vi "S4GUI_003.vi"(7 "Tab ObsEng":enum32{"Obs", "CCD modes", "Guider", "Eng"}(tab)) -> ()   [LabVIEW 2018] (continued)
                n3552 = call-dynamic "Read Interface.vi"("error in (no error)"=w7918, "Channel in"=w7920) -> ("error out"=w7931:errorcluster, "Interface.lvclass"=w7932:refnum<class "Interface.lvclass">, "Channel out"=w7944:refnum<class "Channel.lvclass">)  [unwired: 7 in]
                n3553 = call-dynamic "Write Suffix.vi"("error in (no error)"=w7931, "Suffix"=w7950, "Interface in"=w7932) -> ("error out"=w7949:errorcluster, "Interface out"=w7943:refnum<class "Interface.lvclass">)  [unwired: 7 in]
                n3554 = call-dynamic "Write ObsType.vi"("error in (no error)"=w7949, "ObsType"=w7935, "Interface in"=w7943) -> ("error out"=w7948:errorcluster, "Interface out"=w7942:refnum<class "Interface.lvclass">)  [unwired: 7 in]
                n3555 = call-dynamic "Write Object.vi"("error in (no error)"=w7948, "Object"=w7934, "Interface in"=w7942) -> ("error out"=w7947:errorcluster, "Interface out"=w7941:refnum<class "Interface.lvclass">)  [unwired: 7 in]
                n3556 = call-dynamic "Write Comments.vi"("error in (no error)"=w7947, "Comments"=w7936, "Interface in"=w7941) -> ("error out"=w7930:errorcluster, "Interface out"=w7929:refnum<class "Interface.lvclass">)  [unwired: 7 in]
                n3557 = call-dynamic "Write Observer.vi"("error in (no error)"=w7930, "Observer"=w7933, "Interface in"=w7929) -> ("error out"=w7928:errorcluster, "Interface out"=w7927:refnum<class "Interface.lvclass">)  [unwired: 7 in]
                n3558 = call-dynamic "Write Interface.vi"("error in (no error)"=w7928, "Interface.lvclass"=w7927, "Channel in"=w7944) -> ("error out"=w7924:errorcluster, "Channel out"=w7926:refnum<class "Channel.lvclass">)  [unwired: 7 in]
                n3559 = disable-structure shown="Enabled" {
                  disable-tunnel: w7926 -> [w7961 w7966]
                  disable-tunnel: [w7959 w7966] -> w7925
                  disable-tunnel: w7924 -> [w7958 w7965]
                  disable-tunnel: [w7957 w7965] -> w7923
                  frame Disabled {
                    n3560 = call-dynamic "Read State Machine.vi"("error in (no error)"=w7958, "Device in"=w7961) -> ("error out"=w7964:errorcluster, "State Machine.lvclass"=w7956:refnum<class "State Machine.lvclass">, "Device out"=w7960:refnum<class "Channel.lvclass">)  [unwired: 7 in]
                    n3561 = call "Next State.vi"("error in (no error)"=w7964, "New_State"=12, "State Machine in"=w7956) -> ("error out"=w7963:errorcluster, "State Machine out"=w7955:refnum<class "State Machine.lvclass">)  [unwired: 7 in]
                    n3562 = call-dynamic "Write State Machine.vi"("error in (no error)"=w7963, "State Machine.lvclass"=w7955, "Device in"=w7960) -> ("error out"=w7957:errorcluster, "Device out"=w7959:refnum<class "Channel.lvclass">)  [unwired: 7 in]
                  }
                  frame Enabled {
                  }
                }
                n3563 = call-dynamic "Write Channel.vi"("error in (no error)"=w7923, "Channel.lvclass"=w7925, "Acquisition in"=w7939) -> ("error out"=w7937:errorcluster, "Acquisition out"=w7938:refnum<class "Acquisition.lvclass">)  [unwired: 7 in]
                n3564 = call-dynamic "Write AcquisitionD.vi"("error in (no error)"=w7937, "Acquisition.lvclass"=w7938, "S4ACS_GUI in"=w7940) -> ("error out"=w7951:errorcluster, "S4ACS_GUI out"=w7952:refnum<class "S4GUI.lvclass">)  [unwired: 7 in]
              }
            }
          }
          frame True {
          }
        }
      }
      event "Observer": Mouse Enter {
        n3565 = event-data() -> ()  [unwired: 1 in, 4 out]
        n3566 = disable-structure shown="Disabled" {
          disable-tunnel: [w7974 w7977] -> w7970
          disable-tunnel: w7969 -> [w7972 w7977]
          frame Disabled {
            n3567 = property on="Observer" class="Str"() -> ("Value"=w7973:string)  [unwired: 2 in, 2 out]
            n3568 = String Length(string=w7973) -> (length=w7976:i32)
            n3569 = Equal To 0?(x=w7976) -> (x = 0?=w7975:bool)
            n3570 = property on="Observer" class="Str"(error in=w7972, "Caption.Visible"=w7975) -> (error out=w7974:errorcluster)  [unwired: 1 in, 1 out]
          }
          frame Enabled {
            # "Não se usa mais o texto de fundo\ndo controle \"Observer\""
          }
        }
      }
      event "Filter1", "Filter2", "Filter3", "Filter4": Value Change {
        n3571 = event-data() -> ()  [unwired: 1 in, 6 out]
        n3572 = stacked-sequence {
          seq-local: [w8008 _ _ _] -> [_ w8072 _ _]
          seq-local: [w8007 _ _ _] -> [_ w8071 _ _]
          seq-local: [_ w8070 _ _] -> [_ _ w8121 _]
          seq-local: [_ w8069 _ _] -> [_ _ w8120 _]
          seq-local: [_ _ w8119 _] -> [_ _ _ w8170]
          seq-local: [_ _ w8118 _] -> [_ _ _ w8169]
          tunnel: w7985 -> [w8020 _ _ _]
          tunnel: w7986 -> [w8019 _ _ _]
          tunnel: [_ _ _ w8168] -> w7979
          tunnel: [_ _ _ w8167] -> w7978
          tunnel: w7983 -> [w8006 w8068 w8117 w8166]
          tunnel: w7982 -> [w8005 w8067 w8103 w8152]
          tunnel: w7980 -> [w8004 w8053 w8102 w8151]
          tunnel: w7984 -> [w8003 w8052 w8101 w8150]
          tunnel: w7981 -> [w8002 w8051 w8100 w8149]
          frame #0 {
            # "observer"
            # "comment"
            # "object"
            # "suffix"
            # "obsType"
            n3573 = call-dynamic "Read AcquisitionA.vi"("error in (no error)"=w8020, "S4ACS_GUI in"=w8019) -> ("error out"=w8018:errorcluster, "Acquisition.lvclass"=w8017:refnum<class "Acquisition.lvclass">, "S4ACS_GUI out"=w8012:refnum<class "S4GUI.lvclass">)  [unwired: 7 in]
            n3574 = call-dynamic "Read Channel.vi"("error in (no error)"=w8018, "Acquisition in"=w8017) -> ("error out"=w7988:errorcluster, "Channel.lvclass"=w7991:refnum<class "Channel.lvclass">, "Acquisition out"=w8011:refnum<class "Acquisition.lvclass">)  [unwired: 7 in]
            n3575 = local read "Filter1"() -> (w7989:u8)
            n3576 = call-dynamic "Write Filter.vi"("error in (no error)"=w7988, "Filter"=w7989, "Channel in"=w7991) -> ("error out"=w7987:errorcluster, "Channel out"=w7990:refnum<class "Channel.lvclass">)  [unwired: 7 in]
            n3577 = call-dynamic "Read Interface.vi"("error in (no error)"=w7987, "Channel in"=w7990) -> ("error out"=w7998:errorcluster, "Interface.lvclass"=w7999:refnum<class "Interface.lvclass">, "Channel out"=w8016:refnum<class "Channel.lvclass">)  [unwired: 7 in]
            n3578 = call-dynamic "Write Suffix.vi"("error in (no error)"=w7998, "Suffix"=w8006, "Interface in"=w7999) -> ("error out"=w8023:errorcluster, "Interface out"=w8015:refnum<class "Interface.lvclass">)  [unwired: 7 in]
            n3579 = call-dynamic "Write ObsType.vi"("error in (no error)"=w8023, "ObsType"=w8004, "Interface in"=w8015) -> ("error out"=w8022:errorcluster, "Interface out"=w8014:refnum<class "Interface.lvclass">)  [unwired: 7 in]
            n3580 = call-dynamic "Write Object.vi"("error in (no error)"=w8022, "Object"=w8003, "Interface in"=w8014) -> ("error out"=w8021:errorcluster, "Interface out"=w8013:refnum<class "Interface.lvclass">)  [unwired: 7 in]
            n3581 = call-dynamic "Write Comments.vi"("error in (no error)"=w8021, "Comments"=w8005, "Interface in"=w8013) -> ("error out"=w8001:errorcluster, "Interface out"=w8000:refnum<class "Interface.lvclass">)  [unwired: 7 in]
            n3582 = call-dynamic "Write Observer.vi"("error in (no error)"=w8001, "Observer"=w8002, "Interface in"=w8000) -> ("error out"=w7996:errorcluster, "Interface out"=w7997:refnum<class "Interface.lvclass">)  [unwired: 7 in]
            n3583 = call-dynamic "Write Interface.vi"("error in (no error)"=w7996, "Interface.lvclass"=w7997, "Channel in"=w8016) -> ("error out"=w7993:errorcluster, "Channel out"=w7995:refnum<class "Channel.lvclass">)  [unwired: 7 in]
            n3584 = disable-structure shown="Enabled" {
              disable-tunnel: w7995 -> [w8033 w8035]
              disable-tunnel: [w8031 w8035] -> w7994
              disable-tunnel: w7993 -> [w8030 w8034]
              disable-tunnel: [w8025 w8034] -> w7992
              frame Disabled {
                n3585 = call-dynamic "Read State Machine.vi"("error in (no error)"=w8030, "Device in"=w8033) -> ("error out"=w8029:errorcluster, "State Machine.lvclass"=w8027:refnum<class "State Machine.lvclass">, "Device out"=w8032:refnum<class "Channel.lvclass">)  [unwired: 7 in]
                n3586 = call "Next State.vi"("error in (no error)"=w8029, "New_State"=12, "State Machine in"=w8027) -> ("error out"=w8028:errorcluster, "State Machine out"=w8026:refnum<class "State Machine.lvclass">)  [unwired: 7 in]
                n3587 = call-dynamic "Write State Machine.vi"("error in (no error)"=w8028, "State Machine.lvclass"=w8026, "Device in"=w8032) -> ("error out"=w8025:errorcluster, "Device out"=w8031:refnum<class "Channel.lvclass">)  [unwired: 7 in]
              }
              frame Enabled {
              }
            }
            n3588 = call-dynamic "Write Channel.vi"("error in (no error)"=w7992, "Channel.lvclass"=w7994, "Acquisition in"=w8011) -> ("error out"=w8009:errorcluster, "Acquisition out"=w8010:refnum<class "Acquisition.lvclass">)  [unwired: 7 in]
            n3589 = call-dynamic "Write AcquisitionA.vi"("error in (no error)"=w8009, "Acquisition.lvclass"=w8010, "S4ACS_GUI in"=w8012) -> ("error out"=w8007:errorcluster, "S4ACS_GUI out"=w8008:refnum<class "S4GUI.lvclass">)  [unwired: 7 in]
          }
          frame #1 {
            # "object"
            # "suffix"
            # "obsType"
            n3590 = call "Read AcquisitionB.vi"("error in (no error)"=w8071, "S4ACS_GUI in"=w8072) -> ("error out"=w8057:errorcluster, "Acquisition.lvclass"=w8058:refnum<class "Acquisition.lvclass">, "S4ACS_GUI out"=w8063:refnum<class "S4GUI.lvclass">)  [unwired: 7 in]
            n3591 = call-dynamic "Read Channel.vi"("error in (no error)"=w8057, "Acquisition in"=w8058) -> ("error out"=w8037:errorcluster, "Channel.lvclass"=w8039:refnum<class "Channel.lvclass">, "Acquisition out"=w8064:refnum<class "Acquisition.lvclass">)  [unwired: 7 in]
            n3592 = local read "Filter2"() -> (w8040:u8)
            n3593 = call-dynamic "Write Filter.vi"("error in (no error)"=w8037, "Filter"=w8040, "Channel in"=w8039) -> ("error out"=w8036:errorcluster, "Channel out"=w8038:refnum<class "Channel.lvclass">)  [unwired: 7 in]
            n3594 = call-dynamic "Read Interface.vi"("error in (no error)"=w8036, "Channel in"=w8038) -> ("error out"=w8045:errorcluster, "Interface.lvclass"=w8046:refnum<class "Interface.lvclass">, "Channel out"=w8059:refnum<class "Channel.lvclass">)  [unwired: 7 in]
            n3595 = call-dynamic "Write Suffix.vi"("error in (no error)"=w8045, "Suffix"=w8068, "Interface in"=w8046) -> ("error out"=w8054:errorcluster, "Interface out"=w8060:refnum<class "Interface.lvclass">)  [unwired: 7 in]
            n3596 = call-dynamic "Write ObsType.vi"("error in (no error)"=w8054, "ObsType"=w8053, "Interface in"=w8060) -> ("error out"=w8055:errorcluster, "Interface out"=w8061:refnum<class "Interface.lvclass">)  [unwired: 7 in]
            n3597 = call-dynamic "Write Object.vi"("error in (no error)"=w8055, "Object"=w8052, "Interface in"=w8061) -> ("error out"=w8056:errorcluster, "Interface out"=w8062:refnum<class "Interface.lvclass">)  [unwired: 7 in]
            n3598 = call-dynamic "Write Comments.vi"("error in (no error)"=w8056, "Comments"=w8067, "Interface in"=w8062) -> ("error out"=w8048:errorcluster, "Interface out"=w8047:refnum<class "Interface.lvclass">)  [unwired: 7 in]
            n3599 = call-dynamic "Write Observer.vi"("error in (no error)"=w8048, "Observer"=w8051, "Interface in"=w8047) -> ("error out"=w8049:errorcluster, "Interface out"=w8050:refnum<class "Interface.lvclass">)  [unwired: 7 in]
            n3600 = call-dynamic "Write Interface.vi"("error in (no error)"=w8049, "Interface.lvclass"=w8050, "Channel in"=w8059) -> ("error out"=w8043:errorcluster, "Channel out"=w8044:refnum<class "Channel.lvclass">)  [unwired: 7 in]
            n3601 = disable-structure shown="Enabled" {
              disable-tunnel: w8044 -> [w8077 w8084]
              disable-tunnel: w8043 -> [w8076 w8083]
              disable-tunnel: [w8074 w8084] -> w8042
              disable-tunnel: [w8073 w8083] -> w8041
              frame Disabled {
                n3602 = call-dynamic "Read State Machine.vi"("error in (no error)"=w8076, "Device in"=w8077) -> ("error out"=w8082:errorcluster, "State Machine.lvclass"=w8080:refnum<class "State Machine.lvclass">, "Device out"=w8075:refnum<class "Channel.lvclass">)  [unwired: 7 in]
                n3603 = call "Next State.vi"("error in (no error)"=w8082, "New_State"=12, "State Machine in"=w8080) -> ("error out"=w8081:errorcluster, "State Machine out"=w8079:refnum<class "State Machine.lvclass">)  [unwired: 7 in]
                n3604 = call-dynamic "Write State Machine.vi"("error in (no error)"=w8081, "State Machine.lvclass"=w8079, "Device in"=w8075) -> ("error out"=w8073:errorcluster, "Device out"=w8074:refnum<class "Channel.lvclass">)  [unwired: 7 in]
              }
              frame Enabled {
              }
            }
            n3605 = call-dynamic "Write Channel.vi"("error in (no error)"=w8041, "Channel.lvclass"=w8042, "Acquisition in"=w8064) -> ("error out"=w8066:errorcluster, "Acquisition out"=w8065:refnum<class "Acquisition.lvclass">)  [unwired: 7 in]
            n3606 = call "Write AcquisitionB.vi"("error in (no error)"=w8066, "Acquisition.lvclass"=w8065, "S4ACS_GUI in"=w8063) -> ("error out"=w8069:errorcluster, "S4ACS_GUI out"=w8070:refnum<class "S4GUI.lvclass">)  [unwired: 7 in]
          }
          frame #2 {
            # "object"
            # "suffix"
            # "obsType"
            n3607 = call-dynamic "Read AcquisitionC.vi"("error in (no error)"=w8120, "S4ACS_GUI in"=w8121) -> ("error out"=w8113:errorcluster, "Acquisition.lvclass"=w8112:refnum<class "Acquisition.lvclass">, "S4ACS_GUI out"=w8107:refnum<class "S4GUI.lvclass">)  [unwired: 7 in]
            n3608 = call-dynamic "Read Channel.vi"("error in (no error)"=w8113, "Acquisition in"=w8112) -> ("error out"=w8087:errorcluster, "Channel.lvclass"=w8089:refnum<class "Channel.lvclass">, "Acquisition out"=w8106:refnum<class "Acquisition.lvclass">)  [unwired: 7 in]
            n3609 = local read "Filter3"() -> (w8090:u8)
            n3610 = call-dynamic "Write Filter.vi"("error in (no error)"=w8087, "Filter"=w8090, "Channel in"=w8089) -> ("error out"=w8086:errorcluster, "Channel out"=w8088:refnum<class "Channel.lvclass">)  [unwired: 7 in]
            n3611 = call-dynamic "Read Interface.vi"("error in (no error)"=w8086, "Channel in"=w8088) -> ("error out"=w8098:errorcluster, "Interface.lvclass"=w8099:refnum<class "Interface.lvclass">, "Channel out"=w8111:refnum<class "Channel.lvclass">)  [unwired: 7 in]
            n3612 = call-dynamic "Write Suffix.vi"("error in (no error)"=w8098, "Suffix"=w8117, "Interface in"=w8099) -> ("error out"=w8116:errorcluster, "Interface out"=w8110:refnum<class "Interface.lvclass">)  [unwired: 7 in]
            n3613 = call-dynamic "Write ObsType.vi"("error in (no error)"=w8116, "ObsType"=w8102, "Interface in"=w8110) -> ("error out"=w8115:errorcluster, "Interface out"=w8109:refnum<class "Interface.lvclass">)  [unwired: 7 in]
            n3614 = call-dynamic "Write Object.vi"("error in (no error)"=w8115, "Object"=w8101, "Interface in"=w8109) -> ("error out"=w8114:errorcluster, "Interface out"=w8108:refnum<class "Interface.lvclass">)  [unwired: 7 in]
            n3615 = call-dynamic "Write Comments.vi"("error in (no error)"=w8114, "Comments"=w8103, "Interface in"=w8108) -> ("error out"=w8095:errorcluster, "Interface out"=w8094:refnum<class "Interface.lvclass">)  [unwired: 7 in]
            n3616 = call-dynamic "Write Observer.vi"("error in (no error)"=w8095, "Observer"=w8100, "Interface in"=w8094) -> ("error out"=w8096:errorcluster, "Interface out"=w8097:refnum<class "Interface.lvclass">)  [unwired: 7 in]
            n3617 = call-dynamic "Write Interface.vi"("error in (no error)"=w8096, "Interface.lvclass"=w8097, "Channel in"=w8111) -> ("error out"=w8092:errorcluster, "Channel out"=w8093:refnum<class "Channel.lvclass">)  [unwired: 7 in]
            n3618 = disable-structure shown="Enabled" {
              disable-tunnel: w8093 -> [w8128 w8133]
              disable-tunnel: w8092 -> [w8127 w8132]
              disable-tunnel: [w8122 w8132] -> w8091
              disable-tunnel: [w8125 w8133] -> w8085
              frame Disabled {
                n3619 = call-dynamic "Read State Machine.vi"("error in (no error)"=w8127, "Device in"=w8128) -> ("error out"=w8131:errorcluster, "State Machine.lvclass"=w8124:refnum<class "State Machine.lvclass">, "Device out"=w8126:refnum<class "Channel.lvclass">)  [unwired: 7 in]
                n3620 = call "Next State.vi"("error in (no error)"=w8131, "New_State"=12, "State Machine in"=w8124) -> ("error out"=w8130:errorcluster, "State Machine out"=w8123:refnum<class "State Machine.lvclass">)  [unwired: 7 in]
                n3621 = call-dynamic "Write State Machine.vi"("error in (no error)"=w8130, "State Machine.lvclass"=w8123, "Device in"=w8126) -> ("error out"=w8122:errorcluster, "Device out"=w8125:refnum<class "Channel.lvclass">)  [unwired: 7 in]
              }
              frame Enabled {
              }
            }
            n3622 = call-dynamic "Write Channel.vi"("error in (no error)"=w8091, "Channel.lvclass"=w8085, "Acquisition in"=w8106) -> ("error out"=w8104:errorcluster, "Acquisition out"=w8105:refnum<class "Acquisition.lvclass">)  [unwired: 7 in]
            n3623 = call-dynamic "Write AcquisitionC.vi"("error in (no error)"=w8104, "Acquisition.lvclass"=w8105, "S4ACS_GUI in"=w8107) -> ("error out"=w8118:errorcluster, "S4ACS_GUI out"=w8119:refnum<class "S4GUI.lvclass">)  [unwired: 7 in]
          }
          frame #3 {
            # "object"
            # "suffix"
            # "obsType"
            n3624 = call-dynamic "Read AcquisitionD.vi"("error in (no error)"=w8169, "S4ACS_GUI in"=w8170) -> ("error out"=w8162:errorcluster, "Acquisition.lvclass"=w8161:refnum<class "Acquisition.lvclass">, "S4ACS_GUI out"=w8156:refnum<class "S4GUI.lvclass">)  [unwired: 7 in]
            n3625 = call-dynamic "Read Channel.vi"("error in (no error)"=w8162, "Acquisition in"=w8161) -> ("error out"=w8135:errorcluster, "Channel.lvclass"=w8137:refnum<class "Channel.lvclass">, "Acquisition out"=w8155:refnum<class "Acquisition.lvclass">)  [unwired: 7 in]
            n3626 = local read "Filter4"() -> (w8138:u8)
            n3627 = call-dynamic "Write Filter.vi"("error in (no error)"=w8135, "Filter"=w8138, "Channel in"=w8137) -> ("error out"=w8134:errorcluster, "Channel out"=w8136:refnum<class "Channel.lvclass">)  [unwired: 7 in]
            n3628 = call-dynamic "Read Interface.vi"("error in (no error)"=w8134, "Channel in"=w8136) -> ("error out"=w8147:errorcluster, "Interface.lvclass"=w8148:refnum<class "Interface.lvclass">, "Channel out"=w8160:refnum<class "Channel.lvclass">)  [unwired: 7 in]
            n3629 = call-dynamic "Write Suffix.vi"("error in (no error)"=w8147, "Suffix"=w8166, "Interface in"=w8148) -> ("error out"=w8165:errorcluster, "Interface out"=w8159:refnum<class "Interface.lvclass">)  [unwired: 7 in]
            n3630 = call-dynamic "Write ObsType.vi"("error in (no error)"=w8165, "ObsType"=w8151, "Interface in"=w8159) -> ("error out"=w8164:errorcluster, "Interface out"=w8158:refnum<class "Interface.lvclass">)  [unwired: 7 in]
            n3631 = call-dynamic "Write Object.vi"("error in (no error)"=w8164, "Object"=w8150, "Interface in"=w8158) -> ("error out"=w8163:errorcluster, "Interface out"=w8157:refnum<class "Interface.lvclass">)  [unwired: 7 in]
            n3632 = call-dynamic "Write Comments.vi"("error in (no error)"=w8163, "Comments"=w8152, "Interface in"=w8157) -> ("error out"=w8146:errorcluster, "Interface out"=w8145:refnum<class "Interface.lvclass">)  [unwired: 7 in]
            n3633 = call-dynamic "Write Observer.vi"("error in (no error)"=w8146, "Observer"=w8149, "Interface in"=w8145) -> ("error out"=w8144:errorcluster, "Interface out"=w8143:refnum<class "Interface.lvclass">)  [unwired: 7 in]
            n3634 = call-dynamic "Write Interface.vi"("error in (no error)"=w8144, "Interface.lvclass"=w8143, "Channel in"=w8160) -> ("error out"=w8140:errorcluster, "Channel out"=w8142:refnum<class "Channel.lvclass">)  [unwired: 7 in]
            n3635 = disable-structure shown="Enabled" {
              disable-tunnel: w8142 -> [w8177 w8182]
              disable-tunnel: [w8175 w8182] -> w8141
              disable-tunnel: w8140 -> [w8174 w8181]
              disable-tunnel: [w8173 w8181] -> w8139
              frame Disabled {
                n3636 = call-dynamic "Read State Machine.vi"("error in (no error)"=w8174, "Device in"=w8177) -> ("error out"=w8180:errorcluster, "State Machine.lvclass"=w8172:refnum<class "State Machine.lvclass">, "Device out"=w8176:refnum<class "Channel.lvclass">)  [unwired: 7 in]
                n3637 = call "Next State.vi"("error in (no error)"=w8180, "New_State"=12, "State Machine in"=w8172) -> ("error out"=w8179:errorcluster, "State Machine out"=w8171:refnum<class "State Machine.lvclass">)  [unwired: 7 in]
                n3638 = call-dynamic "Write State Machine.vi"("error in (no error)"=w8179, "State Machine.lvclass"=w8171, "Device in"=w8176) -> ("error out"=w8173:errorcluster, "Device out"=w8175:refnum<class "Channel.lvclass">)  [unwired: 7 in]
              }
              frame Enabled {
              }
            }
            n3639 = call-dynamic "Write Channel.vi"("error in (no error)"=w8139, "Channel.lvclass"=w8141, "Acquisition in"=w8155) -> ("error out"=w8153:errorcluster, "Acquisition out"=w8154:refnum<class "Acquisition.lvclass">)  [unwired: 7 in]
            n3640 = call-dynamic "Write AcquisitionD.vi"("error in (no error)"=w8153, "Acquisition.lvclass"=w8154, "S4ACS_GUI in"=w8156) -> ("error out"=w8167:errorcluster, "S4ACS_GUI out"=w8168:refnum<class "S4GUI.lvclass">)  [unwired: 7 in]
          }
        }
      }
      event "Start ch1": Value Change {
        n3641 = event-data() -> ()  [unwired: 1 in, 6 out]
        n3642 = call "Read Instrument.lvclass.vi"("error in (no error)"=w8195, "S4ACS_GUI in"=w8197) -> ("error out"=w8198:errorcluster, "Instrument.lvclass"=w8199:refnum<class "Instrument.lvclass">, "S4ACS_GUI out"=w8196:refnum<class "S4GUI.lvclass">)  [unwired: 7 in]
        n3643 = call-dynamic "Read mode.vi"("error in (no error)"=w8198, "Instrument in"=w8199) -> ("error out"=w8194:errorcluster, "mode"=w8193:bool)  [unwired: 7 in, 1 out]
        n3644 = call-dynamic "Read AcquisitionA.vi"("error in (no error)"=w8194, "S4ACS_GUI in"=w8196) -> ("error out"=w8211:errorcluster, "Acquisition.lvclass"=w8212:refnum<class "Acquisition.lvclass">, "S4ACS_GUI out"=w8214:refnum<class "S4GUI.lvclass">)  [unwired: 7 in]
        n3645 = call-dynamic "Read Acq_state.vi"("error in (no error)"=w8211, "Acquisition in"=w8212) -> ("error out"=w8208:errorcluster, "Acq_state"=w8210:u32, "Acquisition out"=w8207:refnum<class "Acquisition.lvclass">)  [unwired: 7 in]
        n3646 = Not Equal?(x=w8210, y=u32 400) -> (x != y?=w8213:bool)
        n3647 = case shown="True" w8213 {
          tunnel: w8214 -> [w8227 w8266]
          tunnel: [w8227 w8257] -> w8206
          tunnel: [w8222 w8247] -> w8192
          tunnel: w8208 -> [w8229 w8260]
          tunnel: w8207 -> [w8232 w8256]
          tunnel: [w8223 w8248] -> w8205
          tunnel: w8204 -> [_ w8279]
          tunnel: w8203 -> [_ w8278]
          tunnel: w8202 -> [_ w8277]
          tunnel: w8201 -> [_ w8276]
          tunnel: w8200 -> [_ w8271]
          tunnel: w8193 -> [_ _]
          tunnel: w8191 -> [_ w8251]
          tunnel: w8190 -> [_ w8254]
          tunnel: w8189 -> [_ w8253]
          tunnel: w8188 -> [_ w8252]
          frame False {
            n3648 = call-dynamic "Read Acq_prevstate.vi"("error in (no error)"=w8229, "Acquisition in"=w8232) -> ("error out"=w8228:errorcluster, "Acq_prevstate"=w8230:u32, "Acquisition out"=w8231:refnum<class "Acquisition.lvclass">)  [unwired: 7 in]
            n3649 = call-dynamic "Write Acq_state.vi"("error in (no error)"=w8228, "Acq_state"=w8230, "Acquisition in"=w8231) -> ("error out"=w8219:errorcluster, "Acquisition out"=w8221:refnum<class "Acquisition.lvclass">)  [unwired: 7 in]
            n3650 = call-dynamic "Read enabled.vi"("error in (no error)"=w8219, "Server in"=w8221) -> ("error out"=w8218:errorcluster, "enabled"=w8215:bool, "Server out"=w8220:refnum<class "Acquisition.lvclass">)  [unwired: 7 in]
            n3651 = call-dynamic "Read Channel.vi"("error in (no error)"=w8218, "Acquisition in"=w8220) -> ("error out"=w8216:errorcluster, "Channel.lvclass"=w8217:refnum<class "Channel.lvclass">, "Acquisition out"=w8226:refnum<class "Acquisition.lvclass">)  [unwired: 7 in]
            n3652 = case shown="True" w8215 {
              tunnel: w8217 -> [w8234 w8244]
              tunnel: [w8234 w8242] -> w8225
              tunnel: w8216 -> [w8233 w8239]
              tunnel: [w8233 w8237] -> w8224
              frame False {
              }
              frame True {
                n3653 = call-dynamic "Read State Machine.vi"("error in (no error)"=w8239, "Device in"=w8244) -> ("error out"=w8235:errorcluster, "State Machine.lvclass"=w8236:refnum<class "State Machine.lvclass">, "Device out"=w8243:refnum<class "Channel.lvclass">)  [unwired: 7 in]
                n3654 = call "Next State.vi"("error in (no error)"=w8235, "New_State"=96, "State Machine in"=w8236) -> ("error out"=w8238:errorcluster, "State Machine out"=w8241:refnum<class "State Machine.lvclass">)  [unwired: 7 in]
                n3655 = call-dynamic "Write State Machine.vi"("error in (no error)"=w8238, "State Machine.lvclass"=w8241, "Device in"=w8243) -> ("error out"=w8237:errorcluster, "Device out"=w8242:refnum<class "Channel.lvclass">)  [unwired: 7 in]
              }
            }
            n3656 = call-dynamic "Write Channel.vi"("error in (no error)"=w8224, "Channel.lvclass"=w8225, "Acquisition in"=w8226) -> ("error out"=w8222:errorcluster, "Acquisition out"=w8223:refnum<class "Acquisition.lvclass">)  [unwired: 7 in]
          }
          frame True {
            # "vide S4GUI:\nHandleObservationAsync.vi"
            # "object"
            # "suffix"
            # "obsType"
            n3657 = call "Read Instrument.lvclass.vi"("S4ACS_GUI in"=w8266) -> ("error out"=w8268:errorcluster, "Instrument.lvclass"=w8270:refnum<class "Instrument.lvclass">, "S4ACS_GUI out"=w8258:refnum<class "S4GUI.lvclass">)  [unwired: 8 in]
            n3658 = call "Read WPROT.vi"("error in (no error)"=w8268, "Instrument in"=w8270) -> ("error out"=w8267:errorcluster, "Opt_Selector.lvclass"=w8269:refnum<class "Opt_Selector.lvclass">)  [unwired: 7 in, 1 out]
            n3659 = call-dynamic "Read sequencia.vi"("error in (no error)"=w8267, "Opt_Selector in"=w8269) -> ()  [unwired: 7 in, 3 out]
            n3660 = case shown="\"FOCUS\"" w8251 {
              tunnel: [u32 271 ("Obs_state") u32 251 ("Obs_state")] -> w8259
              tunnel: w8260 -> [w8302 w8313]
              tunnel: [w8301 w8313] -> w8255
              tunnel: w8254 -> [w8309 _]
              tunnel: w8253 -> [w8308 _]
              tunnel: w8252 -> [w8307 _]
              tunnel: w8258 -> [w8300 w8312]
              tunnel: [w8299 w8312] -> w8257
              frame "FOCUS" {
                n3661 = call-dynamic "Read TelFocus.lvclass.vi"("error in (no error)"=w8302, "S4GUI in"=w8300) -> ("error out"=w8304:errorcluster, "TelFocus.lvclass"=w8306:refnum<class "TelFocus.lvclass">, "S4GUI out"=w8310:refnum<class "S4GUI.lvclass">)  [unwired: 7 in]
                n3662 = call-dynamic "LoadParam.vi"("#steps"=w8307, "error in (no error)"=w8304, "step"=w8308, "init"=w8309, "TelFocus in"=w8306) -> ("error out"=w8303:errorcluster, "TelFocus out"=w8305:refnum<class "TelFocus.lvclass">)  [unwired: 5 in]
                n3663 = call-dynamic "Write TelFocus.lvclass.vi"("error in (no error)"=w8303, "TelFocus.lvclass"=w8305, "S4GUI in"=w8310) -> ("error out"=w8301:errorcluster, "S4GUI out"=w8299:refnum<class "S4GUI.lvclass">)  [unwired: 7 in]
              }
              frame Default {
              }
            }
            n3664 = property on="Start ch1" class="Bool"(error in=w8260, "DisabledEnum"=T12."Disabled and Grayed Out" ("Disabled")) -> ()  [unwired: 1 in, 2 out]
            n3665 = call-dynamic "Write Acq_state.vi"("error in (no error)"=w8255, "Acq_state"=w8259, "Acquisition in"=w8256) -> ("error out"=w8280:errorcluster, "Acquisition out"=w8281:refnum<class "Acquisition.lvclass">)  [unwired: 7 in]
            n3666 = call-dynamic "Read Channel.vi"("error in (no error)"=w8280, "Acquisition in"=w8281) -> ("error out"=w8282:errorcluster, "Channel.lvclass"=w8283:refnum<class "Channel.lvclass">, "Acquisition out"=w8287:refnum<class "Acquisition.lvclass">)  [unwired: 7 in]
            n3667 = call-dynamic "Read Interface.vi"("error in (no error)"=w8282, "Channel in"=w8283) -> ("error out"=w8297:errorcluster, "Interface.lvclass"=w8298:refnum<class "Interface.lvclass">, "Channel out"=w8296:refnum<class "Channel.lvclass">)  [unwired: 7 in]
            n3668 = call "Write Exposure Time.vi"("error in (no error)"=w8297, "Exposure Time"="Exptime ch1", "Interface in"=w8298) -> ("error out"=w8264:errorcluster, "Interface out"=w8265:refnum<class "Interface.lvclass">)  [unwired: 7 in]
            n3669 = case shown="Default" w8251 {
              tunnel: w8265 -> [w8316 w8321]
              tunnel: w8264 -> [w8315 w8320]
              tunnel: "Exptime ch1" -> [_ w8319]
              tunnel: [w8315 w8318] -> w8262
              tunnel: [w8316 w8317] -> w8261
              frame "ZERO" {
              }
              frame Default {
                n3670 = call-dynamic "Write prev ExpTime.vi"("error in (no error)"=w8320, "prev ExpTime"=w8319, "Interface in"=w8321) -> ("error out"=w8318:errorcluster, "Interface out"=w8317:refnum<class "Interface.lvclass">)  [unwired: 7 in]
              }
            }
            n3671 = call-dynamic "Write Suffix.vi"("error in (no error)"=w8262, "Suffix"=w8279, "Interface in"=w8261) -> ("error out"=w8295:errorcluster, "Interface out"=w8294:refnum<class "Interface.lvclass">)  [unwired: 7 in]
            n3672 = call-dynamic "Write ObsType.vi"("error in (no error)"=w8295, "ObsType"=w8277, "Interface in"=w8294) -> ("error out"=w8292:errorcluster, "Interface out"=w8293:refnum<class "Interface.lvclass">)  [unwired: 7 in]
            n3673 = call-dynamic "Write Object.vi"("error in (no error)"=w8292, "Object"=w8276, "Interface in"=w8293) -> ("error out"=w8291:errorcluster, "Interface out"=w8290:refnum<class "Interface.lvclass">)  [unwired: 7 in]
            n3674 = call-dynamic "Write Comments.vi"("error in (no error)"=w8291, "Comments"=w8278, "Interface in"=w8290) -> ("error out"=w8288:errorcluster, "Interface out"=w8289:refnum<class "Interface.lvclass">)  [unwired: 7 in]
            n3675 = call-dynamic "Write DS9.vi"("error in (no error)"=w8288, "DS9"="F", "Interface in"=w8289) -> ("error out"=w8273:errorcluster, "Interface out"=w8275:refnum<class "Interface.lvclass">)  [unwired: 7 in]
            n3676 = call-dynamic "Write Observer.vi"("error in (no error)"=w8273, "Observer"=w8271, "Interface in"=w8275) -> ("error out"=w8272:errorcluster, "Interface out"=w8274:refnum<class "Interface.lvclass">)  [unwired: 7 in]
            n3677 = call-dynamic "Write Interface.vi"("error in (no error)"=w8272, "Interface.lvclass"=w8274, "Channel in"=w8296) -> ("error out"=w8245:errorcluster, "Channel out"=w8246:refnum<class "Channel.lvclass">)  [unwired: 7 in]
            n3678 = property on="Exposure Time ch1" class="Slide (strict)"("Scale.Maximum"="Exptime ch1", "Scale.Minimum"=0.0 ("Scale.Range:Minimum")) -> ()  [unwired: 2 in, 2 out]
            n3679 = call-dynamic "Write Channel.vi"("error in (no error)"=w8245, "Channel.lvclass"=w8246, "Acquisition in"=w8287) -> ("error out"=w8249:errorcluster, "Acquisition out"=w8250:refnum<class "Acquisition.lvclass">)  [unwired: 7 in]
            n3680 = call-dynamic "CalcCubeDuration.vi"("error in (no error)"=w8249, "Acquisition in"=w8250) -> ("error out"=w8247:errorcluster, "Acquisition out"=w8248:refnum<class "Acquisition.lvclass">)  [unwired: 8 in]
          }
        }
        n3681 = call-dynamic "Write AcquisitionA.vi"("error in (no error)"=w8192, "Acquisition.lvclass"=w8205, "S4ACS_GUI in"=w8206) -> ("error out"=w8185:errorcluster, "S4ACS_GUI out"=w8186:refnum<class "S4GUI.lvclass">)  [unwired: 7 in]
        n3682 = call-dynamic "Write User Event.vi"("error in (no error)"=w8185, "User Event"="START ASYNC CH1", "S4GUI in"=w8186) -> ("error out"=w8183:errorcluster, "S4GUI out"=w8184:refnum<class "S4GUI.lvclass">)  [unwired: 7 in]
      }
      event "Exp ch1", "Exp ch2", "Exp ch3", "Exp ch4": Value Change {
        n3683 = event-data() -> ()  [unwired: 1 in, 6 out]
        n3684 = call-dynamic "Read AcquisitionA.vi"("error in (no error)"=w8406, "S4ACS_GUI in"=w8407) -> ("error out"=w8396:errorcluster, "Acquisition.lvclass"=w8404:refnum<class "Acquisition.lvclass">, "S4ACS_GUI out"=w8405:refnum<class "S4GUI.lvclass">)  [unwired: 7 in]
        n3685 = call-dynamic "Read Channel.vi"("error in (no error)"=w8396, "Acquisition in"=w8404) -> ("error out"=w8397:errorcluster, "Channel.lvclass"=w8403:refnum<class "Channel.lvclass">, "Acquisition out"=w8402:refnum<class "Acquisition.lvclass">)  [unwired: 7 in]
        n3686 = call-dynamic "Read Interface.vi"("error in (no error)"=w8397, "Channel in"=w8403) -> ("error out"=w8395:errorcluster, "Interface.lvclass"=w8398:refnum<class "Interface.lvclass">, "Channel out"=w8400:refnum<class "Channel.lvclass">)  [unwired: 7 in]
        n3687 = call-dynamic "Write # Images.vi"("error in (no error)"=w8395, "# Images"="Exp ch1", "Interface in"=w8398) -> ("error out"=w8394:errorcluster, "Interface out"=w8391:refnum<class "Interface.lvclass">)  [unwired: 7 in]
        n3688 = call-dynamic "Write #PREV Images.vi"("error in (no error)"=w8394, "#PREV FRAMES"="Exp ch1", "Interface in"=w8391) -> ("error out"=w8393:errorcluster, "Interface out"=w8392:refnum<class "Interface.lvclass">)  [unwired: 7 in]
        n3689 = call-dynamic "Write Interface.vi"("error in (no error)"=w8393, "Interface.lvclass"=w8392, "Channel in"=w8400) -> ("error out"=w8390:errorcluster, "Channel out"=w8399:refnum<class "Channel.lvclass">)  [unwired: 7 in]
        n3690 = property on="Exposures Done ch1" class="Slide (strict)"("Scale.Maximum"="Exp ch1", "Scale.Minimum"=0.0 ("Scale.Range:Minimum")) -> ()  [unwired: 2 in, 2 out]
        n3691 = call-dynamic "Write Channel.vi"("error in (no error)"=w8390, "Channel.lvclass"=w8399, "Acquisition in"=w8402) -> ("error out"=w8389:errorcluster, "Acquisition out"=w8401:refnum<class "Acquisition.lvclass">)  [unwired: 7 in]
        n3692 = call-dynamic "Write AcquisitionA.vi"("error in (no error)"=w8389, "Acquisition.lvclass"=w8401, "S4ACS_GUI in"=w8405) -> ("error out"=w8331:errorcluster, "S4ACS_GUI out"=w8332:refnum<class "S4GUI.lvclass">)  [unwired: 7 in]
        n3693 = call "Read AcquisitionB.vi"("error in (no error)"=w8331, "S4ACS_GUI in"=w8332) -> ("error out"=w8378:errorcluster, "Acquisition.lvclass"=w8386:refnum<class "Acquisition.lvclass">, "S4ACS_GUI out"=w8387:refnum<class "S4GUI.lvclass">)  [unwired: 7 in]
        n3694 = call-dynamic "Read Channel.vi"("error in (no error)"=w8378, "Acquisition in"=w8386) -> ("error out"=w8379:errorcluster, "Channel.lvclass"=w8385:refnum<class "Channel.lvclass">, "Acquisition out"=w8384:refnum<class "Acquisition.lvclass">)  [unwired: 7 in]
        n3695 = call-dynamic "Read Interface.vi"("error in (no error)"=w8379, "Channel in"=w8385) -> ("error out"=w8377:errorcluster, "Interface.lvclass"=w8380:refnum<class "Interface.lvclass">, "Channel out"=w8382:refnum<class "Channel.lvclass">)  [unwired: 7 in]
        n3696 = call-dynamic "Write # Images.vi"("error in (no error)"=w8377, "# Images"="Exp ch2", "Interface in"=w8380) -> ("error out"=w8376:errorcluster, "Interface out"=w8373:refnum<class "Interface.lvclass">)  [unwired: 7 in]
        n3697 = call-dynamic "Write #PREV Images.vi"("error in (no error)"=w8376, "#PREV FRAMES"="Exp ch2", "Interface in"=w8373) -> ("error out"=w8375:errorcluster, "Interface out"=w8374:refnum<class "Interface.lvclass">)  [unwired: 7 in]
        n3698 = property on="Exposures Done ch2" class="Slide (strict)"("Scale.Maximum"="Exp ch2", "Scale.Minimum"=0.0 ("Scale.Range:Minimum")) -> ()  [unwired: 2 in, 2 out]
        n3699 = call-dynamic "Write Interface.vi"("error in (no error)"=w8375, "Interface.lvclass"=w8374, "Channel in"=w8382) -> ("error out"=w8372:errorcluster, "Channel out"=w8381:refnum<class "Channel.lvclass">)  [unwired: 7 in]
        n3700 = call-dynamic "Write Channel.vi"("error in (no error)"=w8372, "Channel.lvclass"=w8381, "Acquisition in"=w8384) -> ("error out"=w8371:errorcluster, "Acquisition out"=w8383:refnum<class "Acquisition.lvclass">)  [unwired: 7 in]
        n3701 = call "Write AcquisitionB.vi"("error in (no error)"=w8371, "Acquisition.lvclass"=w8383, "S4ACS_GUI in"=w8387) -> ("error out"=w8333:errorcluster, "S4ACS_GUI out"=w8334:refnum<class "S4GUI.lvclass">)  [unwired: 7 in]
        n3702 = call-dynamic "Read AcquisitionC.vi"("error in (no error)"=w8333, "S4ACS_GUI in"=w8334) -> ("error out"=w8361:errorcluster, "Acquisition.lvclass"=w8369:refnum<class "Acquisition.lvclass">, "S4ACS_GUI out"=w8370:refnum<class "S4GUI.lvclass">)  [unwired: 7 in]
        n3703 = call-dynamic "Read Channel.vi"("error in (no error)"=w8361, "Acquisition in"=w8369) -> ("error out"=w8362:errorcluster, "Channel.lvclass"=w8368:refnum<class "Channel.lvclass">, "Acquisition out"=w8367:refnum<class "Acquisition.lvclass">)  [unwired: 7 in]
        n3704 = call-dynamic "Read Interface.vi"("error in (no error)"=w8362, "Channel in"=w8368) -> ("error out"=w8360:errorcluster, "Interface.lvclass"=w8363:refnum<class "Interface.lvclass">, "Channel out"=w8365:refnum<class "Channel.lvclass">)  [unwired: 7 in]
        n3705 = call-dynamic "Write # Images.vi"("error in (no error)"=w8360, "# Images"="Exp ch3", "Interface in"=w8363) -> ("error out"=w8359:errorcluster, "Interface out"=w8356:refnum<class "Interface.lvclass">)  [unwired: 7 in]
        n3706 = call-dynamic "Write #PREV Images.vi"("error in (no error)"=w8359, "#PREV FRAMES"="Exp ch3", "Interface in"=w8356) -> ("error out"=w8358:errorcluster, "Interface out"=w8357:refnum<class "Interface.lvclass">)  [unwired: 7 in]
        n3707 = call-dynamic "Write Interface.vi"("error in (no error)"=w8358, "Interface.lvclass"=w8357, "Channel in"=w8365) -> ("error out"=w8355:errorcluster, "Channel out"=w8364:refnum<class "Channel.lvclass">)  [unwired: 7 in]
        n3708 = property on="Exposures Done ch3" class="Slide (strict)"("Scale.Maximum"="Exp ch3", "Scale.Minimum"=0.0 ("Scale.Range:Minimum")) -> ()  [unwired: 2 in, 2 out]
        n3709 = call-dynamic "Write Channel.vi"("error in (no error)"=w8355, "Channel.lvclass"=w8364, "Acquisition in"=w8367) -> ("error out"=w8354:errorcluster, "Acquisition out"=w8366:refnum<class "Acquisition.lvclass">)  [unwired: 7 in]
        n3710 = call-dynamic "Write AcquisitionC.vi"("error in (no error)"=w8354, "Acquisition.lvclass"=w8366, "S4ACS_GUI in"=w8370) -> ("error out"=w8335:errorcluster, "S4ACS_GUI out"=w8336:refnum<class "S4GUI.lvclass">)  [unwired: 7 in]
        n3711 = call-dynamic "Read AcquisitionD.vi"("error in (no error)"=w8335, "S4ACS_GUI in"=w8336) -> ("error out"=w8344:errorcluster, "Acquisition.lvclass"=w8352:refnum<class "Acquisition.lvclass">, "S4ACS_GUI out"=w8353:refnum<class "S4GUI.lvclass">)  [unwired: 7 in]
        n3712 = call-dynamic "Read Channel.vi"("error in (no error)"=w8344, "Acquisition in"=w8352) -> ("error out"=w8345:errorcluster, "Channel.lvclass"=w8351:refnum<class "Channel.lvclass">, "Acquisition out"=w8350:refnum<class "Acquisition.lvclass">)  [unwired: 7 in]
        n3713 = call-dynamic "Read Interface.vi"("error in (no error)"=w8345, "Channel in"=w8351) -> ("error out"=w8343:errorcluster, "Interface.lvclass"=w8346:refnum<class "Interface.lvclass">, "Channel out"=w8348:refnum<class "Channel.lvclass">)  [unwired: 7 in]
        n3714 = call-dynamic "Write # Images.vi"("error in (no error)"=w8343, "# Images"="Exp ch4", "Interface in"=w8346) -> ("error out"=w8342:errorcluster, "Interface out"=w8339:refnum<class "Interface.lvclass">)  [unwired: 7 in]
        n3715 = call-dynamic "Write #PREV Images.vi"("error in (no error)"=w8342, "#PREV FRAMES"="Exp ch4", "Interface in"=w8339) -> ("error out"=w8341:errorcluster, "Interface out"=w8340:refnum<class "Interface.lvclass">)  [unwired: 7 in]
        n3716 = call-dynamic "Write Interface.vi"("error in (no error)"=w8341, "Interface.lvclass"=w8340, "Channel in"=w8348) -> ("error out"=w8338:errorcluster, "Channel out"=w8347:refnum<class "Channel.lvclass">)  [unwired: 7 in]
        n3717 = property on="Exposures Done ch4" class="Slide (strict)"("Scale.Maximum"="Exp ch4", "Scale.Minimum"=0.0 ("Scale.Range:Minimum")) -> ()  [unwired: 2 in, 2 out]
        n3718 = call-dynamic "Write Channel.vi"("error in (no error)"=w8338, "Channel.lvclass"=w8347, "Acquisition in"=w8350) -> ("error out"=w8337:errorcluster, "Acquisition out"=w8349:refnum<class "Acquisition.lvclass">)  [unwired: 7 in]
        n3719 = call-dynamic "Write AcquisitionD.vi"("error in (no error)"=w8337, "Acquisition.lvclass"=w8349, "S4ACS_GUI in"=w8353) -> ("error out"=w8329:errorcluster, "S4ACS_GUI out"=w8330:refnum<class "S4GUI.lvclass">)  [unwired: 7 in]
      }
      event "#cycles ch1": Value Change {
        n3720 = event-data() -> ("NewVal"=w8408:u32)  [unwired: 1 in]
        n3721 = call-dynamic "Read AcquisitionA.vi"("error in (no error)"=w8430, "S4ACS_GUI in"=w8431) -> ("error out"=w8425:errorcluster, "Acquisition.lvclass"=w8428:refnum<class "Acquisition.lvclass">, "S4ACS_GUI out"=w8429:refnum<class "S4GUI.lvclass">)  [unwired: 7 in]
        n3722 = call-dynamic "Read Channel.vi"("error in (no error)"=w8425, "Acquisition in"=w8428) -> ("error out"=w8422:errorcluster, "Channel.lvclass"=w8421:refnum<class "Channel.lvclass">, "Acquisition out"=w8427:refnum<class "Acquisition.lvclass">)  [unwired: 7 in]
        n3723 = call-dynamic "Write ciclos.vi"("error in (no error)"=w8422, "ciclos"=w8408, "Channel in"=w8421) -> ("error out"=w8419:errorcluster, "Channel out"=w8420:refnum<class "Channel.lvclass">)  [unwired: 7 in]
        n3724 = call-dynamic "Write prev ciclos.vi"("error in (no error)"=w8419, "prev ciclos"=w8408, "Channel in"=w8420) -> ("error out"=w8417:errorcluster, "Channel out"=w8418:refnum<class "Channel.lvclass">)  [unwired: 7 in]
        n3725 = property on="Cycles Done ch1" class="Slide (strict)"("Scale.Maximum"=w8408, "Scale.Minimum"=0.0 ("Scale.Range:Minimum")) -> ()  [unwired: 2 in, 2 out]
        n3726 = call-dynamic "Write Channel.vi"("error in (no error)"=w8417, "Channel.lvclass"=w8418, "Acquisition in"=w8427) -> ("error out"=w8424:errorcluster, "Acquisition out"=w8426:refnum<class "Acquisition.lvclass">)  [unwired: 7 in]
        n3727 = call-dynamic "Write AcquisitionA.vi"("error in (no error)"=w8424, "Acquisition.lvclass"=w8426, "S4ACS_GUI in"=w8429) -> ("error out"=w8415:errorcluster, "S4ACS_GUI out"=w8416:refnum<class "S4GUI.lvclass">)  [unwired: 7 in]
        n3728 = call-dynamic "Write ciclos.vi"("error in (no error)"=w8415, "ciclos"=w8408, "S4ACS_GUI in"=w8416) -> ("error out"=w8410:errorcluster, "S4ACS_GUI out"=w8412:refnum<class "S4GUI.lvclass">)  [unwired: 7 in]
        n3729 = call-dynamic "Write prev sequencias.vi"("error in (no error)"=w8410, "prev sequencias"=w8408, "S4GUI in"=w8412) -> ("error out"=w8409:errorcluster, "S4GUI out"=w8411:refnum<class "S4GUI.lvclass">)  [unwired: 7 in]
        n3730 = call-dynamic "Write TotalCiclos.vi"("error in (no error)"=w8409, "TotalCiclos"=w8408, "S4GUI in"=w8411) -> ("error out"=w8413:errorcluster, "S4GUI out"=w8414:refnum<class "S4GUI.lvclass">)  [unwired: 7 in]
      }
      event "#cycles ch2": Value Change {
        n3731 = event-data() -> ("NewVal"=w8432:u32)  [unwired: 1 in]
        n3732 = call "Read AcquisitionB.vi"("error in (no error)"=w8454, "S4ACS_GUI in"=w8455) -> ("error out"=w8449:errorcluster, "Acquisition.lvclass"=w8452:refnum<class "Acquisition.lvclass">, "S4ACS_GUI out"=w8453:refnum<class "S4GUI.lvclass">)  [unwired: 7 in]
        n3733 = call-dynamic "Read Channel.vi"("error in (no error)"=w8449, "Acquisition in"=w8452) -> ("error out"=w8447:errorcluster, "Channel.lvclass"=w8446:refnum<class "Channel.lvclass">, "Acquisition out"=w8451:refnum<class "Acquisition.lvclass">)  [unwired: 7 in]
        n3734 = call-dynamic "Write ciclos.vi"("error in (no error)"=w8447, "ciclos"=w8432, "Channel in"=w8446) -> ("error out"=w8444:errorcluster, "Channel out"=w8445:refnum<class "Channel.lvclass">)  [unwired: 7 in]
        n3735 = call-dynamic "Write prev ciclos.vi"("error in (no error)"=w8444, "prev ciclos"=w8432, "Channel in"=w8445) -> ("error out"=w8442:errorcluster, "Channel out"=w8443:refnum<class "Channel.lvclass">)  [unwired: 7 in]
        n3736 = call-dynamic "Write Channel.vi"("error in (no error)"=w8442, "Channel.lvclass"=w8443, "Acquisition in"=w8451) -> ("error out"=w8448:errorcluster, "Acquisition out"=w8450:refnum<class "Acquisition.lvclass">)  [unwired: 7 in]
        n3737 = property on="Cycles Done ch2" class="Slide (strict)"("Scale.Maximum"=w8432, "Scale.Minimum"=0.0 ("Scale.Range:Minimum")) -> ()  [unwired: 2 in, 2 out]
        n3738 = call "Write AcquisitionB.vi"("error in (no error)"=w8448, "Acquisition.lvclass"=w8450, "S4ACS_GUI in"=w8453) -> ("error out"=w8440:errorcluster, "S4ACS_GUI out"=w8441:refnum<class "S4GUI.lvclass">)  [unwired: 7 in]
        n3739 = call-dynamic "Write ciclos.vi"("error in (no error)"=w8440, "ciclos"=w8432, "S4ACS_GUI in"=w8441) -> ("error out"=w8435:errorcluster, "S4ACS_GUI out"=w8437:refnum<class "S4GUI.lvclass">)  [unwired: 7 in]
        n3740 = call-dynamic "Write prev sequencias.vi"("error in (no error)"=w8435, "prev sequencias"=w8432, "S4GUI in"=w8437) -> ("error out"=w8434:errorcluster, "S4GUI out"=w8436:refnum<class "S4GUI.lvclass">)  [unwired: 7 in]
        n3741 = call-dynamic "Write TotalCiclos.vi"("error in (no error)"=w8434, "TotalCiclos"=w8432, "S4GUI in"=w8436) -> ("error out"=w8438:errorcluster, "S4GUI out"=w8439:refnum<class "S4GUI.lvclass">)  [unwired: 7 in]
      }
      event "#cycles ch3": Value Change {
        n3742 = event-data() -> ("NewVal"=w8456:u32)  [unwired: 1 in]
        n3743 = call-dynamic "Read AcquisitionC.vi"("error in (no error)"=w8478, "S4ACS_GUI in"=w8479) -> ("error out"=w8473:errorcluster, "Acquisition.lvclass"=w8476:refnum<class "Acquisition.lvclass">, "S4ACS_GUI out"=w8477:refnum<class "S4GUI.lvclass">)  [unwired: 7 in]
        n3744 = call-dynamic "Read Channel.vi"("error in (no error)"=w8473, "Acquisition in"=w8476) -> ("error out"=w8471:errorcluster, "Channel.lvclass"=w8470:refnum<class "Channel.lvclass">, "Acquisition out"=w8475:refnum<class "Acquisition.lvclass">)  [unwired: 7 in]
        n3745 = call-dynamic "Write ciclos.vi"("error in (no error)"=w8471, "ciclos"=w8456, "Channel in"=w8470) -> ("error out"=w8468:errorcluster, "Channel out"=w8469:refnum<class "Channel.lvclass">)  [unwired: 7 in]
        n3746 = call-dynamic "Write prev ciclos.vi"("error in (no error)"=w8468, "prev ciclos"=w8456, "Channel in"=w8469) -> ("error out"=w8466:errorcluster, "Channel out"=w8467:refnum<class "Channel.lvclass">)  [unwired: 7 in]
        n3747 = call-dynamic "Write Channel.vi"("error in (no error)"=w8466, "Channel.lvclass"=w8467, "Acquisition in"=w8475) -> ("error out"=w8472:errorcluster, "Acquisition out"=w8474:refnum<class "Acquisition.lvclass">)  [unwired: 7 in]
        n3748 = property on="Cycles Done ch3" class="Slide (strict)"("Scale.Maximum"=w8456, "Scale.Minimum"=0.0 ("Scale.Range:Minimum")) -> ()  [unwired: 2 in, 2 out]
        n3749 = call-dynamic "Write AcquisitionC.vi"("error in (no error)"=w8472, "Acquisition.lvclass"=w8474, "S4ACS_GUI in"=w8477) -> ("error out"=w8464:errorcluster, "S4ACS_GUI out"=w8465:refnum<class "S4GUI.lvclass">)  [unwired: 7 in]
        n3750 = call-dynamic "Write ciclos.vi"("error in (no error)"=w8464, "ciclos"=w8456, "S4ACS_GUI in"=w8465) -> ("error out"=w8459:errorcluster, "S4ACS_GUI out"=w8461:refnum<class "S4GUI.lvclass">)  [unwired: 7 in]
        n3751 = call-dynamic "Write prev sequencias.vi"("error in (no error)"=w8459, "prev sequencias"=w8456, "S4GUI in"=w8461) -> ("error out"=w8458:errorcluster, "S4GUI out"=w8460:refnum<class "S4GUI.lvclass">)  [unwired: 7 in]
        n3752 = call-dynamic "Write TotalCiclos.vi"("error in (no error)"=w8458, "TotalCiclos"=w8456, "S4GUI in"=w8460) -> ("error out"=w8462:errorcluster, "S4GUI out"=w8463:refnum<class "S4GUI.lvclass">)  [unwired: 7 in]
      }
      event "#cycles ch4": Value Change {
        n3753 = event-data() -> ("NewVal"=w8480:u32)  [unwired: 1 in]
        n3754 = call-dynamic "Read AcquisitionD.vi"("error in (no error)"=w8502, "S4ACS_GUI in"=w8503) -> ("error out"=w8497:errorcluster, "Acquisition.lvclass"=w8500:refnum<class "Acquisition.lvclass">, "S4ACS_GUI out"=w8501:refnum<class "S4GUI.lvclass">)  [unwired: 7 in]
        n3755 = call-dynamic "Read Channel.vi"("error in (no error)"=w8497, "Acquisition in"=w8500) -> ("error out"=w8495:errorcluster, "Channel.lvclass"=w8494:refnum<class "Channel.lvclass">, "Acquisition out"=w8499:refnum<class "Acquisition.lvclass">)  [unwired: 7 in]
        n3756 = call-dynamic "Write ciclos.vi"("error in (no error)"=w8495, "ciclos"=w8480, "Channel in"=w8494) -> ("error out"=w8492:errorcluster, "Channel out"=w8493:refnum<class "Channel.lvclass">)  [unwired: 7 in]
        n3757 = call-dynamic "Write prev ciclos.vi"("error in (no error)"=w8492, "prev ciclos"=w8480, "Channel in"=w8493) -> ("error out"=w8490:errorcluster, "Channel out"=w8491:refnum<class "Channel.lvclass">)  [unwired: 7 in]
        n3758 = call-dynamic "Write Channel.vi"("error in (no error)"=w8490, "Channel.lvclass"=w8491, "Acquisition in"=w8499) -> ("error out"=w8496:errorcluster, "Acquisition out"=w8498:refnum<class "Acquisition.lvclass">)  [unwired: 7 in]
        n3759 = call-dynamic "Write AcquisitionD.vi"("error in (no error)"=w8496, "Acquisition.lvclass"=w8498, "S4ACS_GUI in"=w8501) -> ("error out"=w8488:errorcluster, "S4ACS_GUI out"=w8489:refnum<class "S4GUI.lvclass">)  [unwired: 7 in]
        n3760 = property on="Cycles Done ch4" class="Slide (strict)"("Scale.Maximum"=w8480, "Scale.Minimum"=0.0 ("Scale.Range:Minimum")) -> ()  [unwired: 2 in, 2 out]
        n3761 = call-dynamic "Write ciclos.vi"("error in (no error)"=w8488, "ciclos"=w8480, "S4ACS_GUI in"=w8489) -> ("error out"=w8483:errorcluster, "S4ACS_GUI out"=w8485:refnum<class "S4GUI.lvclass">)  [unwired: 7 in]
        n3762 = call-dynamic "Write prev sequencias.vi"("error in (no error)"=w8483, "prev sequencias"=w8480, "S4GUI in"=w8485) -> ("error out"=w8482:errorcluster, "S4GUI out"=w8484:refnum<class "S4GUI.lvclass">)  [unwired: 7 in]
        n3763 = call-dynamic "Write TotalCiclos.vi"("error in (no error)"=w8482, "TotalCiclos"=w8480, "S4GUI in"=w8484) -> ("error out"=w8486:errorcluster, "S4GUI out"=w8487:refnum<class "S4GUI.lvclass">)  [unwired: 7 in]
      }
      event "Start ch2": Value Change {
        n3764 = event-data() -> ()  [unwired: 1 in, 6 out]
        n3765 = call "Read Instrument.lvclass.vi"("error in (no error)"=w8517, "S4ACS_GUI in"=w8518) -> ("error out"=w8519:errorcluster, "Instrument.lvclass"=w8520:refnum<class "Instrument.lvclass">, "S4ACS_GUI out"=w8516:refnum<class "S4GUI.lvclass">)  [unwired: 7 in]
        n3766 = call-dynamic "Read mode.vi"("error in (no error)"=w8519, "Instrument in"=w8520) -> ("error out"=w8515:errorcluster, "mode"=w8514:bool)  [unwired: 7 in, 1 out]
        n3767 = call "Read AcquisitionB.vi"("error in (no error)"=w8515, "S4ACS_GUI in"=w8516) -> ("error out"=w8532:errorcluster, "Acquisition.lvclass"=w8533:refnum<class "Acquisition.lvclass">, "S4ACS_GUI out"=w8535:refnum<class "S4GUI.lvclass">)  [unwired: 7 in]
        n3768 = call-dynamic "Read Acq_state.vi"("error in (no error)"=w8532, "Acquisition in"=w8533) -> ("error out"=w8529:errorcluster, "Acq_state"=w8531:u32, "Acquisition out"=w8528:refnum<class "Acquisition.lvclass">)  [unwired: 7 in]
        n3769 = Not Equal?(x=w8531, y=u32 400) -> (x != y?=w8534:bool)
        n3770 = case shown="True" w8534 {
          tunnel: w8535 -> [w8548 w8587]
          tunnel: [w8548 w8579] -> w8527
          tunnel: [w8543 w8569] -> w8513
          tunnel: w8529 -> [w8550 w8577]
